vi "InAngle.vi"(6 "Function":enum16{"Posit", "Merge"}(ring), 7 "Angle":dbl=15.0, 8 "Towards Target?":bool, 9 "2nd Array (Start)":cluster{"X":dbl, "Y":dbl, "Z":dbl}[](array[cluster]), 10 "Base Array (End)":cluster{"X":dbl, "Y":dbl, "Z":dbl}[](array[cluster])) -> (2 "In Angle?":bool=TRUE)   [LabVIEW 2014]
panel:
  out "XY Graph":cluster{dbl[], dbl[]}[](graph)=[{[1.0, 2.0], [1.0, 3.0]}, {[3.0, 4.0], [4.0, 6.0]}]
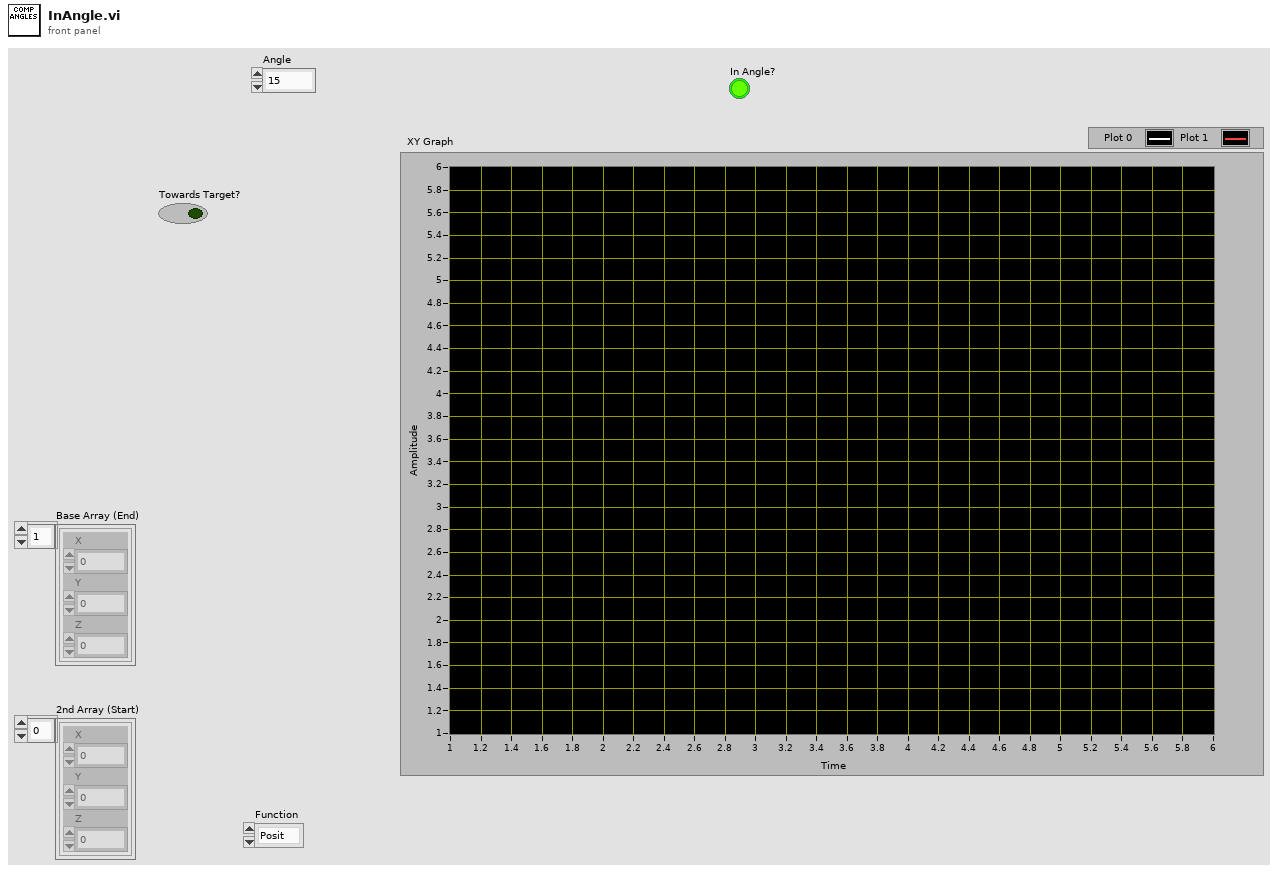
[diagram p1: front panel]
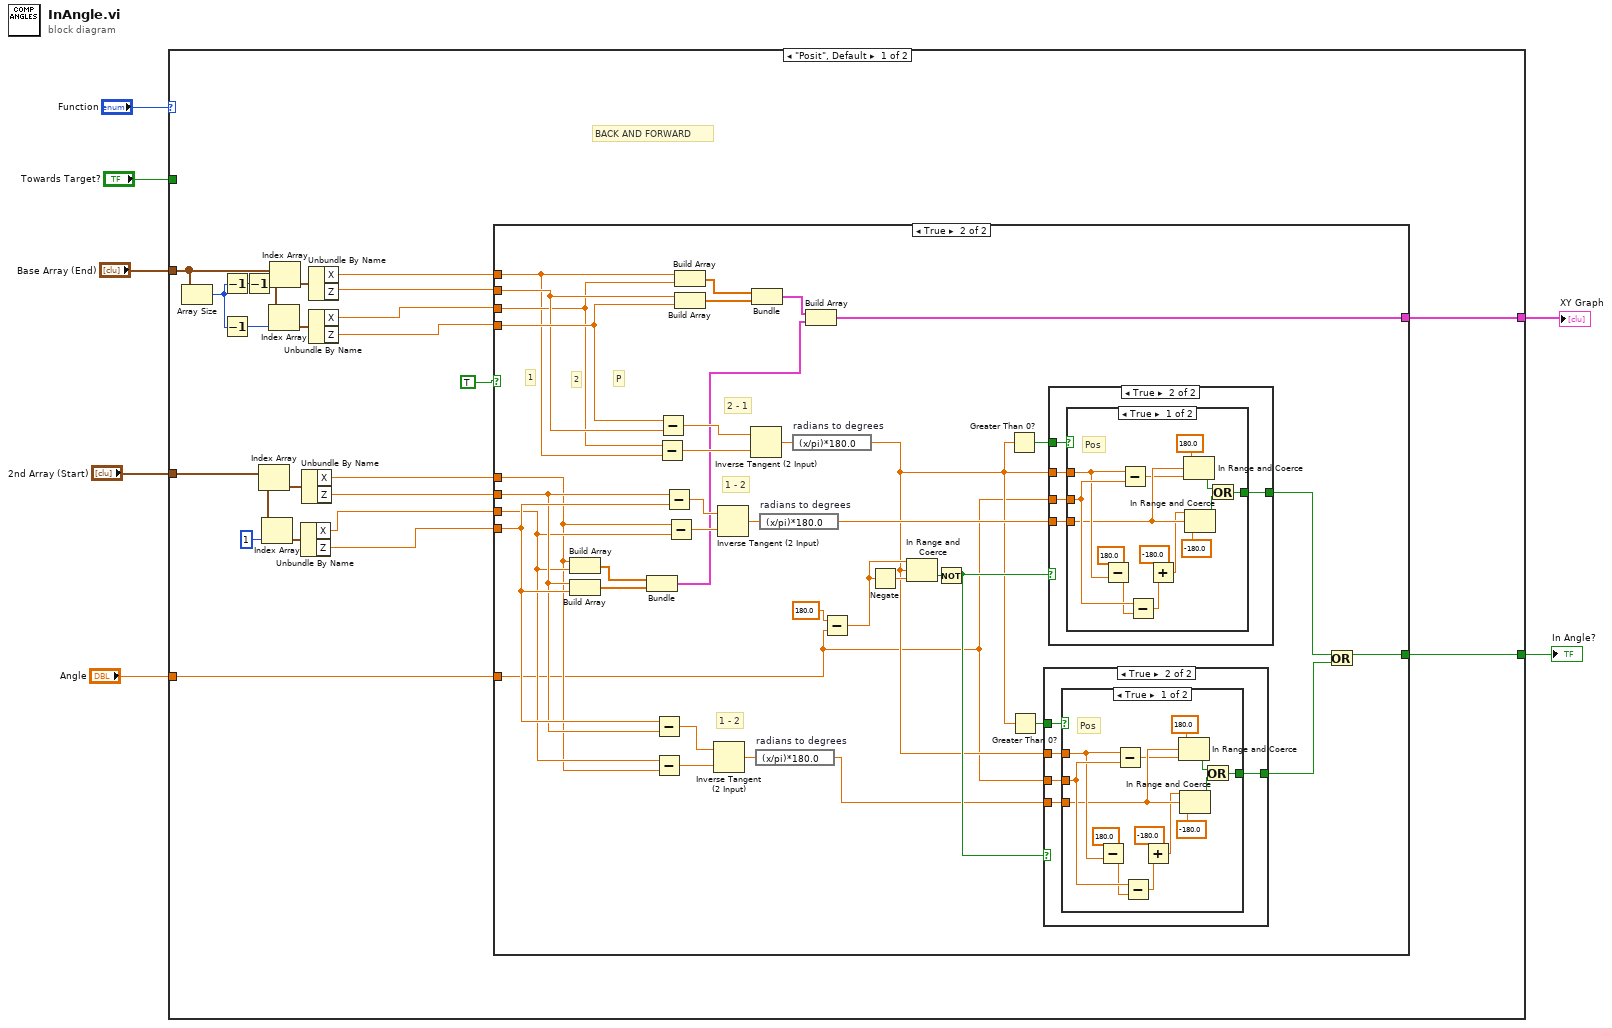
[diagram p0: block diagram]
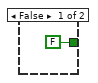
[diagram p2: hidden frame]
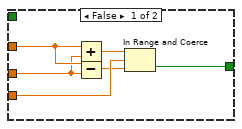
[diagram p3: hidden frame]
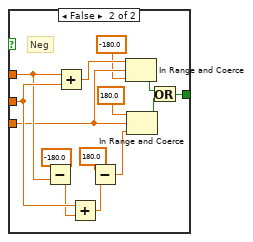
[diagram p4: hidden frame]
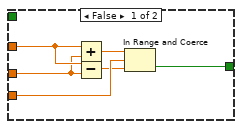
[diagram p5: hidden frame]
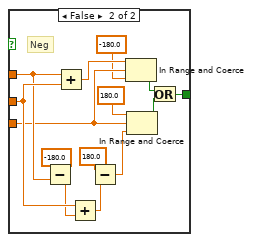
[diagram p6: hidden frame]
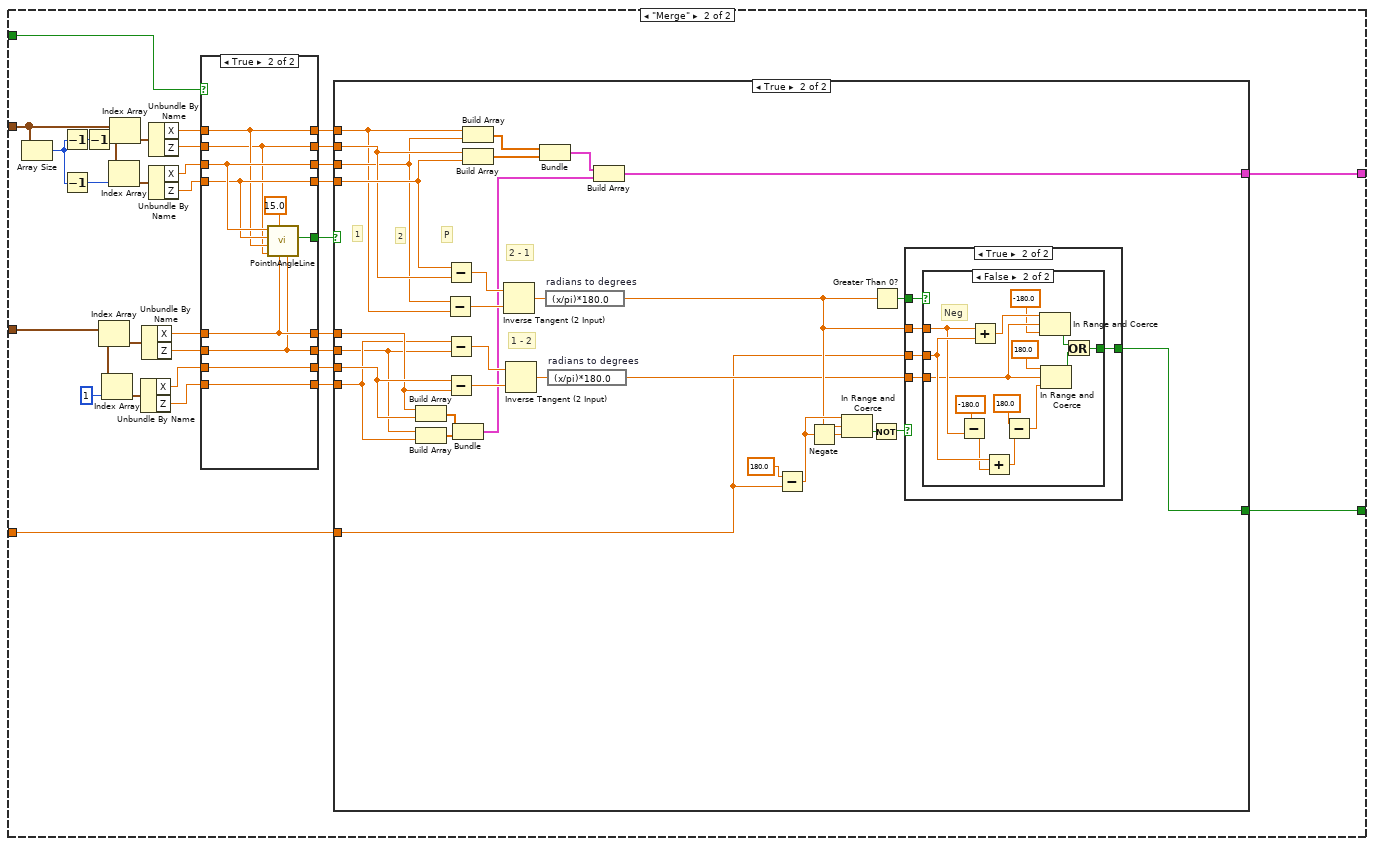
[diagram p7: hidden frame]
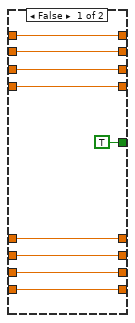
[diagram p8: hidden frame]
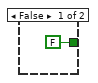
[diagram p9: hidden frame]
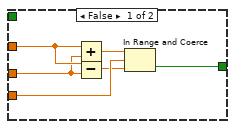
[diagram p10: hidden frame]
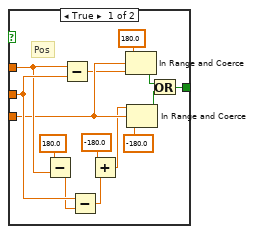
[diagram p11: hidden frame]
diagram:
  n1 = case shown="\"Posit\", Default" "Function" {
    tunnel: [w30 w179] -> w7
    tunnel: "2nd Array (Start)" -> [w28 w178]
    tunnel: "Base Array (End)" -> [w26 w176]
    tunnel: "Angle" -> [w9 w167]
    tunnel: [w8 w166] -> w2
    tunnel: "Towards Target?" -> [_ w149]
    frame "Posit", Default {
      # "BACK AND FORWARD"
      n2 = Array Size(array=w26) -> (size(s)=w25:i32)
      n3 = Decrement(x=w25) -> (x-1=w24:i32)
      n4 = Decrement(x=w25) -> (x-1=w19:i32)
      n5 = Decrement(x=w24) -> (x-1=w18:i32)
      n6 = Index Array(array=w28) -> (element=w22:cluster{"X":dbl, "Y":dbl, "Z":dbl})  [unwired: 1 in]
      n7 = Index Array(array=w28, index=1) -> (element=w23:cluster{"X":dbl, "Y":dbl, "Z":dbl})
      n8 = Index Array(array=w26, index=w19) -> (element=w21:cluster{"X":dbl, "Y":dbl, "Z":dbl})
      n9 = Index Array(array=w26, index=w18) -> (element=w20:cluster{"X":dbl, "Y":dbl, "Z":dbl})
      n10 = Unbundle By Name(w23) -> ("X"=w11:dbl, "Z"=w10:dbl)
      n11 = Unbundle By Name(w22) -> ("X"=w13:dbl, "Z"=w12:dbl)
      n12 = Unbundle By Name(w20) -> ("X"=w17:dbl, "Z"=w16:dbl)
      n13 = Unbundle By Name(w21) -> ("X"=w15:dbl, "Z"=w14:dbl)
      n14 = case shown="True" TRUE {
        tunnel: w17 -> [_ w47]
        tunnel: w16 -> [_ w49]
        tunnel: w15 -> [_ w48]
        tunnel: w14 -> [_ w55]
        tunnel: [FALSE w37] -> w30
        tunnel: w13 -> [_ w39]
        tunnel: w12 -> [_ w41]
        tunnel: w11 -> [_ w40]
        tunnel: w10 -> [_ w42]
        tunnel: w9 -> [_ w32]
        tunnel: [_ w46] -> w8
        frame False {
        }
        frame True {
          # "1 - 2"
          # "P"
          # "2"
          # "1"
          # "1 - 2"
          # "2 - 1"
          n15 = Build Array(w39, w40) -> (w51:dbl[])
          n16 = Build Array(w41, w42) -> (w52:dbl[])
          n17 = Bundle(w51, w52) -> (w50:cluster{dbl[], dbl[]})  [unwired: 1 in]
          n18 = Subtract(x=w42, y=w41) -> (x-y=w45:dbl)
          n19 = Subtract(x=w40, y=w39) -> (x-y=w44:dbl)
          n20 = Subtract(x=w48, y=w47) -> (x-y=w65:dbl)
          n21 = Subtract(x=w55, y=w49) -> (x-y=w64:dbl)
          n22 = Subtract(x=w41, y=w42) -> (x-y=w63:dbl)
          n23 = Subtract(x=w39, y=w40) -> (x-y=w62:dbl)
          n24 = Build Array(w47, w48) -> (w69:dbl[])
          n25 = Build Array(w49, w55) -> (w68:dbl[])
          n26 = Inverse Tangent (2 Input)(1:w44, 2:w45) -> (0:w43:dbl)
          n27 = Inverse Tangent (2 Input)(1:w62, 2:w63) -> (0:w61:dbl)
          n28 = Inverse Tangent (2 Input)(1:w65, 2:w64) -> (0:w66:dbl)
          n29 = Bundle(w69, w68) -> (w67:cluster{dbl[], dbl[]})  [unwired: 1 in]
          n30 = expression code="(x/pi)*180.0" "radians to degrees"(w43) -> (w33:dbl)
          n31 = expression code="(x/pi)*180.0" "radians to degrees"(w61) -> (w54:dbl)
          n32 = expression code="(x/pi)*180.0" "radians to degrees"(w66) -> (w34:dbl)
          n33 = Build Array(w67, w50) -> (w46:cluster{dbl[], dbl[]}[])
          n34 = Subtract(x=180.0, y=w32) -> (x-y=w58:dbl)
          n35 = Negate(x=w58) -> (-x=w59:dbl)
          n36 = In Range and Coerce(upper limit=w58, x=w34, lower limit=w59) -> (In Range?=w57:bool)  [unwired: 1 out]
          n37 = Not(x=w57) -> (.not. x?=w35:bool)
          n38 = Greater Than 0?(x=w34) -> (x > 0?=w56:bool)
          n39 = Greater Than 0?(x=w34) -> (x > 0?=w38:bool)
          n40 = case shown="True" w35 {
            tunnel: w33 -> [w75 w77]
            tunnel: [w72 w79] -> w36
            tunnel: w34 -> [w71 w76]
            tunnel: w32 -> [w70 w78]
            tunnel: w38 -> [_ w80]
            frame False {
              n41 = Add(x=w71, y=w70) -> (x+y=w74:dbl)
              n42 = Subtract(x=w71, y=w70) -> (x-y=w73:dbl)
              n43 = In Range and Coerce(upper limit=w74, x=w75, lower limit=w73) -> (In Range?=w72:bool)  [unwired: 1 out]
            }
            frame True {
              n44 = case shown="True" w80 {
                tunnel: [w89 w103] -> w79
                tunnel: w78 -> [w93 w107]
                tunnel: w77 -> [w85 w99]
                tunnel: w76 -> [w86 w100]
                frame True {
                  # "Pos"
                  n45 = Subtract(x=180.0, y=w86) -> (x-y=w92:dbl)
                  n46 = Subtract(x=w86, y=w93) -> (x-y=w84:dbl)
                  n47 = Subtract(x=w93, y=w92) -> (x-y=w90:dbl)
                  n48 = Add(x=-180.0, y=w90) -> (x+y=w82:dbl)
                  n49 = In Range and Coerce(upper limit=180.0, x=w85, lower limit=w84) -> (In Range?=w87:bool)  [unwired: 1 out]
                  n50 = In Range and Coerce(upper limit=w82, x=w85, lower limit=-180.0) -> (In Range?=w88:bool)  [unwired: 1 out]
                  n51 = Or(x=w87, y=w88) -> (x .or. y?=w89:bool)
                }
                frame False {
                  # "Neg"
                  n52 = Subtract(x=-180.0, y=w100) -> (x-y=w106:dbl)
                  n53 = Add(x=w100, y=w107) -> (x+y=w98:dbl)
                  n54 = Add(x=w107, y=w106) -> (x+y=w104:dbl)
                  n55 = Subtract(x=180.0, y=w104) -> (x-y=w96:dbl)
                  n56 = In Range and Coerce(upper limit=w98, x=w99, lower limit=-180.0) -> (In Range?=w101:bool)  [unwired: 1 out]
                  n57 = In Range and Coerce(upper limit=180.0, x=w99, lower limit=w96) -> (In Range?=w102:bool)  [unwired: 1 out]
                  n58 = Or(x=w101, y=w102) -> (x .or. y?=w103:bool)
                }
              }
            }
          }
          n59 = case shown="True" w35 {
            tunnel: w54 -> [w114 w116]
            tunnel: [w111 w118] -> w53
            tunnel: w34 -> [w110 w115]
            tunnel: w32 -> [w109 w117]
            tunnel: w56 -> [_ w119]
            frame False {
              n60 = Add(x=w110, y=w109) -> (x+y=w113:dbl)
              n61 = Subtract(x=w110, y=w109) -> (x-y=w112:dbl)
              n62 = In Range and Coerce(upper limit=w113, x=w114, lower limit=w112) -> (In Range?=w111:bool)  [unwired: 1 out]
            }
            frame True {
              n63 = case shown="True" w119 {
                tunnel: [w128 w142] -> w118
                tunnel: w117 -> [w132 w146]
                tunnel: w116 -> [w124 w138]
                tunnel: w115 -> [w125 w139]
                frame True {
                  # "Pos"
                  n64 = Subtract(x=180.0, y=w125) -> (x-y=w131:dbl)
                  n65 = Subtract(x=w125, y=w132) -> (x-y=w123:dbl)
                  n66 = Subtract(x=w132, y=w131) -> (x-y=w129:dbl)
                  n67 = Add(x=-180.0, y=w129) -> (x+y=w121:dbl)
                  n68 = In Range and Coerce(upper limit=180.0, x=w124, lower limit=w123) -> (In Range?=w126:bool)  [unwired: 1 out]
                  n69 = In Range and Coerce(upper limit=w121, x=w124, lower limit=-180.0) -> (In Range?=w127:bool)  [unwired: 1 out]
                  n70 = Or(x=w126, y=w127) -> (x .or. y?=w128:bool)
                }
                frame False {
                  # "Neg"
                  n71 = Subtract(x=-180.0, y=w139) -> (x-y=w145:dbl)
                  n72 = Add(x=w139, y=w146) -> (x+y=w137:dbl)
                  n73 = Add(x=w146, y=w145) -> (x+y=w143:dbl)
                  n74 = Subtract(x=180.0, y=w143) -> (x-y=w135:dbl)
                  n75 = In Range and Coerce(upper limit=w137, x=w138, lower limit=-180.0) -> (In Range?=w140:bool)  [unwired: 1 out]
                  n76 = In Range and Coerce(upper limit=180.0, x=w138, lower limit=w135) -> (In Range?=w141:bool)  [unwired: 1 out]
                  n77 = Or(x=w140, y=w141) -> (x .or. y?=w142:bool)
                }
              }
            }
          }
          n78 = Or(x=w53, y=w36) -> (x .or. y?=w37:bool)
        }
      }
    }
    frame "Merge" {
      n79 = Array Size(array=w176) -> (size(s)=w175:i32)
      n80 = Decrement(x=w175) -> (x-1=w174:i32)
      n81 = Decrement(x=w175) -> (x-1=w169:i32)
      n82 = Decrement(x=w174) -> (x-1=w168:i32)
      n83 = Index Array(array=w178) -> (element=w172:cluster{"X":dbl, "Y":dbl, "Z":dbl})  [unwired: 1 in]
      n84 = Index Array(array=w178, index=1) -> (element=w173:cluster{"X":dbl, "Y":dbl, "Z":dbl})
      n85 = Index Array(array=w176, index=w169) -> (element=w171:cluster{"X":dbl, "Y":dbl, "Z":dbl})
      n86 = Index Array(array=w176, index=w168) -> (element=w170:cluster{"X":dbl, "Y":dbl, "Z":dbl})
      n87 = Unbundle By Name(w173) -> ("X"=w163:dbl, "Z"=w164:dbl)
      n88 = Unbundle By Name(w172) -> ("X"=w159:dbl, "Z"=w161:dbl)
      n89 = Unbundle By Name(w170) -> ("X"=w151:dbl, "Z"=w153:dbl)
      n90 = Unbundle By Name(w171) -> ("X"=w155:dbl, "Z"=w156:dbl)
      n91 = case shown="True" w149 {
        tunnel: [w180 w198] -> w165
        tunnel: w164 -> [w180 w198]
        tunnel: w163 -> [w181 w197]
        tunnel: [w181 w197] -> w162
        tunnel: w161 -> [w182 w190]
        tunnel: [w182 w190] -> w160
        tunnel: w159 -> [w183 w191]
        tunnel: [w183 w191] -> w158
        tunnel: w156 -> [w188 w194]
        tunnel: [w188 w194] -> w157
        tunnel: w155 -> [w187 w195]
        tunnel: [w187 w195] -> w154
        tunnel: w153 -> [w186 w192]
        tunnel: [w186 w192] -> w152
        tunnel: w151 -> [w185 w193]
        tunnel: [w185 w193] -> w150
        tunnel: [TRUE ("In Angle?") w196] -> w148
        frame False {
        }
        frame True {
          n92 = call "PointInAngleLine.vi"("PointY"=w190, "PointX"=w191, "Angle (D: 10)"=15.0, "Line2Y"=w192, "Line2X"=w193, "Line1Y"=w194, "Line1X"=w195) -> ("In Angle?"=w196:bool)  [unwired: 4 in]
        }
      }
      n93 = case shown="True" w148 {
        tunnel: w150 -> [_ w205]
        tunnel: w152 -> [_ w208]
        tunnel: w154 -> [_ w207]
        tunnel: w157 -> [_ w214]
        tunnel: [FALSE w212] -> w179
        tunnel: w158 -> [_ w203]
        tunnel: w160 -> [_ w201]
        tunnel: w162 -> [_ w204]
        tunnel: w165 -> [_ w202]
        tunnel: w167 -> [_ w206]
        tunnel: [_ w200] -> w166
        frame False {
        }
        frame True {
          # "P"
          # "2"
          # "1"
          # "1 - 2"
          # "2 - 1"
          n94 = Build Array(w203, w204) -> (w210:dbl[])
          n95 = Build Array(w201, w202) -> (w211:dbl[])
          n96 = Subtract(x=w207, y=w205) -> (x-y=w226:dbl)
          n97 = Subtract(x=w214, y=w208) -> (x-y=w225:dbl)
          n98 = Subtract(x=w202, y=w201) -> (x-y=w224:dbl)
          n99 = Subtract(x=w204, y=w203) -> (x-y=w223:dbl)
          n100 = Bundle(w210, w211) -> (w209:cluster{dbl[], dbl[]})  [unwired: 1 in]
          n101 = Build Array(w205, w207) -> (w230:dbl[])
          n102 = Build Array(w208, w214) -> (w229:dbl[])
          n103 = Inverse Tangent (2 Input)(1:w226, 2:w225) -> (0:w227:dbl)
          n104 = Inverse Tangent (2 Input)(1:w223, 2:w224) -> (0:w222:dbl)
          n105 = Bundle(w230, w229) -> (w228:cluster{dbl[], dbl[]})  [unwired: 1 in]
          n106 = expression code="(x/pi)*180.0" "radians to degrees"(w227) -> (w215:dbl)
          n107 = expression code="(x/pi)*180.0" "radians to degrees"(w222) -> (w213:dbl)
          n108 = Build Array(w228, w209) -> (w200:cluster{dbl[], dbl[]}[])
          n109 = Subtract(x=180.0, y=w206) -> (x-y=w219:dbl)
          n110 = Negate(x=w219) -> (-x=w220:dbl)
          n111 = In Range and Coerce(upper limit=w219, x=w215, lower limit=w220) -> (In Range?=w218:bool)  [unwired: 1 out]
          n112 = Not(x=w218) -> (.not. x?=w217:bool)
          n113 = Greater Than 0?(x=w215) -> (x > 0?=w216:bool)
          n114 = case shown="True" w217 {
            tunnel: w213 -> [w236 w238]
            tunnel: [w233 w240] -> w212
            tunnel: w215 -> [w232 w237]
            tunnel: w206 -> [w231 w239]
            tunnel: w216 -> [_ w241]
            frame False {
              n115 = Add(x=w232, y=w231) -> (x+y=w235:dbl)
              n116 = Subtract(x=w232, y=w231) -> (x-y=w234:dbl)
              n117 = In Range and Coerce(upper limit=w235, x=w236, lower limit=w234) -> (In Range?=w233:bool)  [unwired: 1 out]
            }
            frame True {
              n118 = case shown="False" w241 {
                tunnel: [w250 w264] -> w240
                tunnel: w239 -> [w254 w268]
                tunnel: w238 -> [w246 w260]
                tunnel: w237 -> [w247 w261]
                frame True {
                  # "Pos"
                  n119 = Subtract(x=180.0, y=w247) -> (x-y=w253:dbl)
                  n120 = Subtract(x=w247, y=w254) -> (x-y=w245:dbl)
                  n121 = Subtract(x=w254, y=w253) -> (x-y=w251:dbl)
                  n122 = Add(x=-180.0, y=w251) -> (x+y=w243:dbl)
                  n123 = In Range and Coerce(upper limit=180.0, x=w246, lower limit=w245) -> (In Range?=w248:bool)  [unwired: 1 out]
                  n124 = In Range and Coerce(upper limit=w243, x=w246, lower limit=-180.0) -> (In Range?=w249:bool)  [unwired: 1 out]
                  n125 = Or(x=w248, y=w249) -> (x .or. y?=w250:bool)
                }
                frame False {
                  # "Neg"
                  n126 = Subtract(x=-180.0, y=w261) -> (x-y=w267:dbl)
                  n127 = Add(x=w261, y=w268) -> (x+y=w259:dbl)
                  n128 = Add(x=w268, y=w267) -> (x+y=w265:dbl)
                  n129 = Subtract(x=180.0, y=w265) -> (x-y=w257:dbl)
                  n130 = In Range and Coerce(upper limit=w259, x=w260, lower limit=-180.0) -> (In Range?=w262:bool)  [unwired: 1 out]
                  n131 = In Range and Coerce(upper limit=180.0, x=w260, lower limit=w257) -> (In Range?=w263:bool)  [unwired: 1 out]
                  n132 = Or(x=w262, y=w263) -> (x .or. y?=w264:bool)
                }
              }
            }
          }
        }
      }
    }
  }
  "In Angle?" <- w7
  "XY Graph" <- w2
